vi "testRemoveComments.vi"(8 "error in (no error)":errorcluster, 11 "reference in":refnum<class "EasyXMLTest.lvclass">) -> (0 "error out":errorcluster, 3 "reference in":refnum<class "EasyXMLTest.lvclass">)   [LabVIEW 2013, in "EasyXMLTest.lvclass"]
uses:
  EasyXMLTest.lvclass
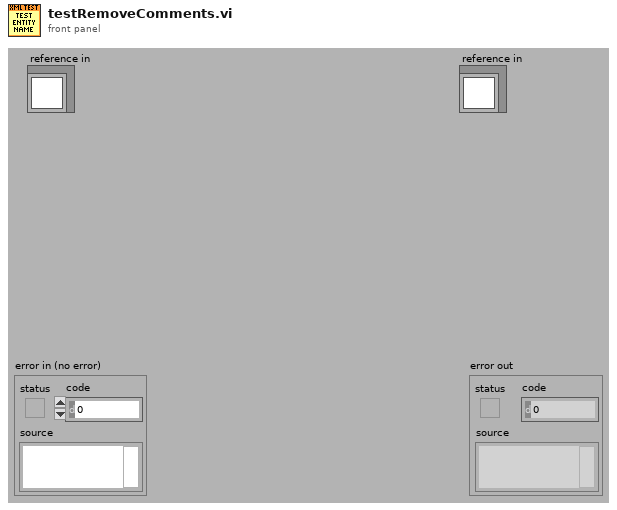
[diagram p1: front panel]
types:
  T1 = cluster{"SubEntities":cluster{"Entity":cluster{"#attributes":cluster{"foo":string}}}}
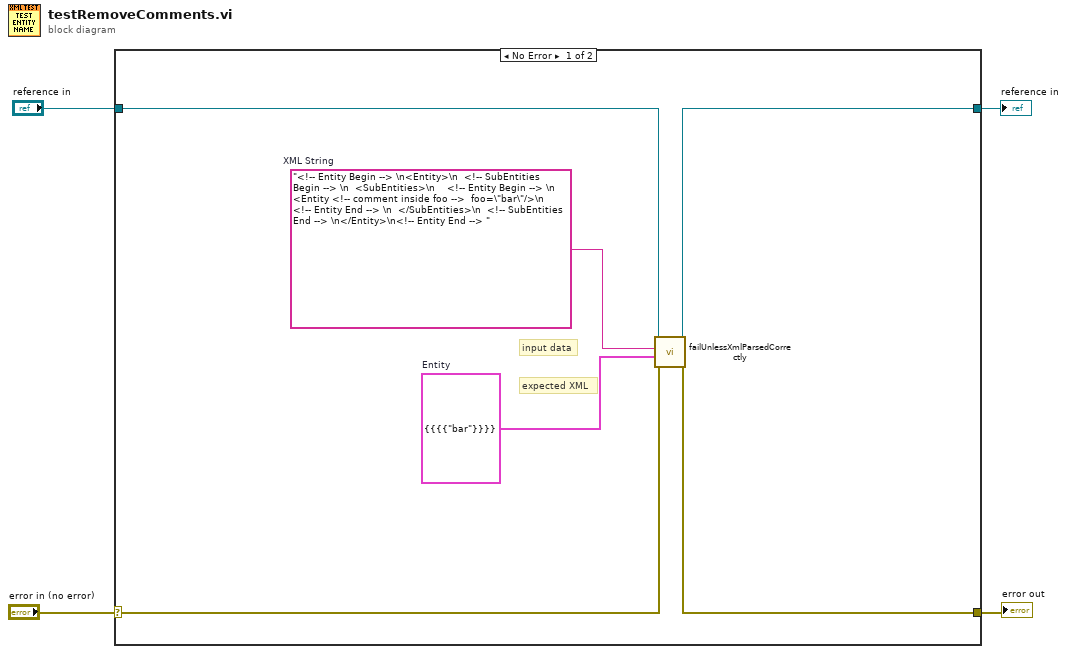
[diagram p0: block diagram]
diagram:
  n1 = case shown="No Error" "error in (no error)" {
    selector: "error in (no error)" -> [w7 w12]
    tunnel: [w10 w12] -> w3
    tunnel: [w8 w11] -> w1
    tunnel: "reference in" -> [w9 w11]
    frame No Error {
      w5 = T1 {"SubEntities"={"Entity"={"#attributes"={"foo"="bar"}}}}  # Entity
      w6 = "<!-- Entity Begin --> \n<Entity>\n  <!-- SubEntities Begin --> \n  <SubEntities>\n    <!-- Entity Begin --> \n    <Entity <!-- comment inside foo -->  foo=\"bar\"/>\n    <!-- Entity End --> \n  </SubEntities>\n  <!-- SubEntities End --> \n</Entity>\n<!-- Entity End --> "  # XML String
      # "expected XML"
      # "input data"
      n2 = call "failUnlessXmlParsedCorrectly.vi"("error in"=w7, "Expected Data"=w5, "XML String"=w6, "reference in"=w9) -> ("error out"=w10:errorcluster, "reference in"=w8:refnum<class "EasyXMLTest.lvclass">)  [unwired: 5 in, 1 out]
    }
    frame Error {
    }
  }
  "error out" <- w3
  "reference in" <- w1
